vi "Current VI Path - EXE Aware.vi"(4 "Current VI's Path in":path) -> (1 "Current VI's Path (EXE Aware)":path)   [LabVIEW 2023]
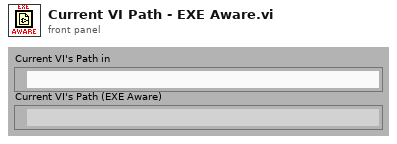
[diagram p1: front panel]
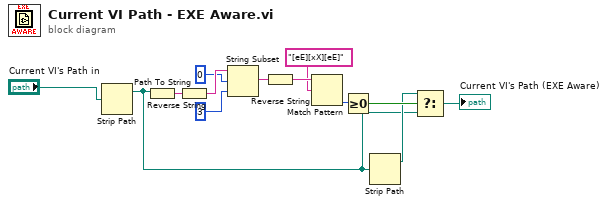
[diagram p0: block diagram]
diagram:
  n1 = Strip Path(path="Current VI's Path in") -> (stripped path=w3:path)  [unwired: 1 out]
  n2 = Path To String(path=w3) -> (string=w13:string)
  n3 = Reverse String(1:w13) -> (0:w12:string)
  n4 = String Subset(string=w12, offset (0)=0, length (rest)=3 ("length")) -> (substring=w9:string)
  n5 = Reverse String(1:w9) -> (0:w8:string)
  n6 = Match Pattern(string=w8, regular expression="[eE][xX][eE]") -> (offset past match=w6:i32)  [unwired: 1 in, 3 out]
  n7 = Greater Or Equal To 0?(x=w6) -> (x >= 0?=w5:bool)
  n8 = Strip Path(path=w3) -> (stripped path=w4:path)  [unwired: 1 out]
  n9 = Select(t=w4, s=w5, f=w3) -> (s? t:f=→"Current VI's Path (EXE Aware)":path)
